vi "CalculateAverages.vi"(6 "Settings":T1={"Name of test"="", "Date"=timestamp(0 s since 1904-01-01), "Location"="", "Template"="", "Soundcard"="", "resolution"=32, "Sampling rate"=48000, "Ch1 Gain "=25.0, "Ch2 Gain"=10.0, "Sample time (s)"=0.3, "Pre-trigger (s)"=0.01, "Hammer Threshold"=10.0, "Positions"=12, "Taps/Position"=5, "Set Names"="", "Freq resolution"=10.0, "Hammer cutoff"=0.0, "Mic cutoff"=0.0, "Double bounce "=0.0, "Hammer Cal"=10.0, "dB Offset"=0.0, "Accel Cal"=10.0, "Vibrometer Cal"=0.0, "Mic Cal"=0.0, "Output"=2, "Voltage Cal"=1.0, "Vibrometer Port"="ASRL27::INSTR", "Range"=4, "High Pass"=2, "Bandwidth"=4, "X Range"=[], "Y Range"=[], "dB Spread"=0.0, "Trigger"=0, "Ch_1"=25, "Ch_2"=25, "flip?"=FALSE, "60Hz"=FALSE, "Time offset"=0.0, "Piezo Cal"=1.0, "Default Notes"=""} {"Ch_2" min=1 step=1; "Ch_1" min=1 max=100 step=1; "Trigger" items=["Hammer (force)", "Self-tap", "Spacebar"]; "Bandwidth" items=["1 kHz"=1, "5 kHz"=5, "10 kHz"=10, "25 kHz"=25, "50 kHz"=50, "100 kHz"=100]; "High Pass" items=["Off", "13 Hz", "104 Hz"]; "Range" items=["10 mm/s"=1, "20 mm/s"=2, "50 mm/s"=5, "100 mm/s"=10, "200 mm/s"=20, "500 mm/s"=50, "1 m/s"=100, "2 m/s"=200]; "Output" items=["Accelerometer", "Speed (from acceleration)", "Microphone", "Vibrometer", "Piezo"]; "Voltage Cal" format="%#_13g"; "Ch2 Gain" format="%#_13g"; "Ch1 Gain" format="%#_13g"; "Double bounce" min=0.0; "Mic cutoff" min=0.0 format="%#_4g"; "Hammer cutoff" min=0.0 format="%#_4g"; "Freq resolution" min=0.0; "Pre-trigger (s)" format="%#_13g"; "Date" format="%<%H:%M\n%d/%m/%y>T"; "resolution" items=["16 bit"=16, "24 bit"=24, "32 bit"=32]; "Sampling rate" items=["22050 samp/s"=22050, "44100 samp/s"=44100, "48000 samp/s"=48000]}, 8 "Task":enum16{"Set", "Test"}(ring), 10 "Inst:Test Name":string, 11 "Last Data File":path) -> ()   [LabVIEW 2022 SP3]
uses:
  PreferencesControl.ctl
panel:
  # "Hz"
  # "dB"
  # "dB"
  # "sec"
  # "sec"
  # "mV/Pa"
  # "mV/m/s2"
  # "mV/mm/s"
  # "V/N"
  # "sec"
  # "sec"
  # "mV/N"
  # "a.u."
  # "a.u."
  # "sec"
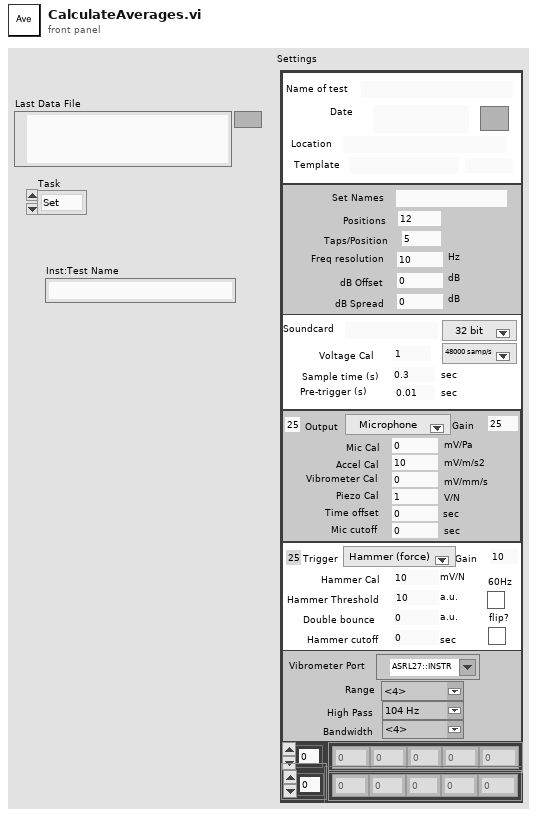
[diagram p1: front panel]
types:
  T1 = typedef "PreferencesControl.ctl" = cluster{"Name of test":string, "Date":timestamp, "Location":string, "Template":string, "Soundcard":string, "resolution":u16, "Sampling rate":u16, "Ch1 Gain ":dbl, "Ch2 Gain":dbl, "Sample time (s)":dbl, "Pre-trigger (s)":dbl, "Hammer Threshold":dbl, "Positions":i16, "Taps/Position":i16, "Set Names":string, "Freq resolution":dbl, "Hammer cutoff":dbl, "Mic cutoff":dbl, "Double bounce ":dbl, "Hammer Cal":dbl, "dB Offset":dbl, "Accel Cal":dbl, "Vibrometer Cal":dbl, "Mic Cal":dbl, "Output":u16, "Voltage Cal":dbl, "Vibrometer Port":refnum<visa-resource-name>, "Range":u16, "High Pass":u16, "Bandwidth":u16, "X Range":cluster{"Minimum":dbl, "Maximum":dbl, "Increment":dbl, "Minor Increment":dbl, "Start":dbl}[], "Y Range":cluster{"Minimum":dbl, "Maximum":dbl, "Increment":dbl, "Minor Increment":dbl, "Start":dbl}[], "dB Spread":dbl, "Trigger":u16, "Ch_1":u8, "Ch_2":u8, "flip?":bool, "60Hz":bool, "Time offset":dbl, "Piezo Cal":dbl, "Default Notes":string}
  T2 = cluster{"Test":string, "Set":string, "Position":string, "Tap":string}
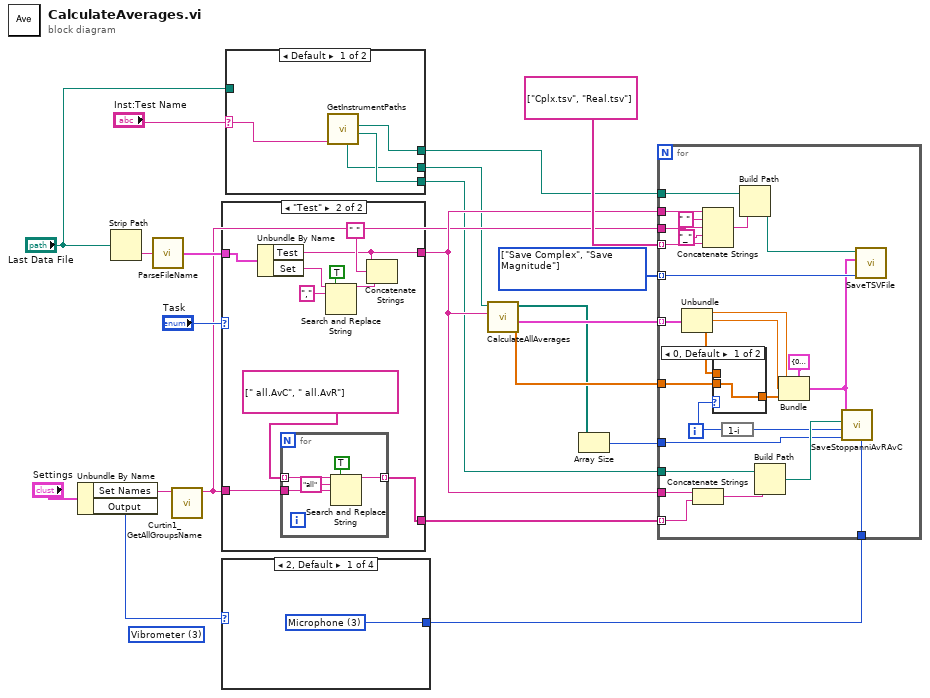
[diagram p0: block diagram]
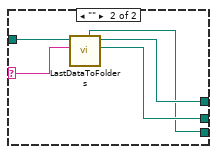
[diagram p2: hidden frame]
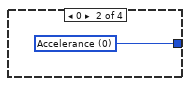
[diagram p3: hidden frame]
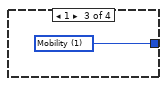
[diagram p4: hidden frame]
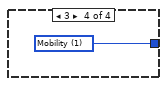
[diagram p5: hidden frame]
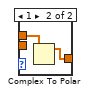
[diagram p6: hidden frame]
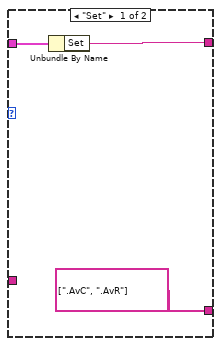
[diagram p7: hidden frame]
diagram:
  w7 = enum16{"Save Magnitude", "Save Complex"}[] [enum."Save Complex", enum."Save Magnitude"] items=["Save Magnitude", "Save Complex"]
  (unwired) u16 3 items=["Acclerometer", "Displacement", "Microphone", "Vibrometer"] ("Channel 1")
  n1 = Unbundle By Name("Settings") -> ("Set Names"=w12:string, "Output"=w9:u16)
  n2 = Strip Path(path="Last Data File") -> (name=w21:string)  [unwired: 1 out]
  n3 = call "ParseFileName.vi"("String in"=w21) -> ("Name"=w18:T2)  [unwired: 2 out]
  n4 = call "Curtin1_GetAllGroupsName.vi"("Set Names in"=w12) -> ("Set Names out"=w6:string)  [unwired: 10 in]
  n5 = case shown="\"Test\"" "Task" {
    tunnel: w18 -> [w24 w34]
    tunnel: [w23 w28] -> w15
    tunnel: [string[] [".AvC", ".AvR"] w26] -> w14
    tunnel: w6 -> [_ w25]
    frame "Set" {
      n6 = Unbundle By Name(w24) -> ("Set"=w23:string)
    }
    frame "Test" {
      n7 = Unbundle By Name(w34) -> ("Test"=w28:string, "Set"=w32:string)
      n8 = for {
        tunnel: string[] [" all.AvC", " all.AvR"] -> [w38] mode=indexing
        tunnel: [w37] -> w26 mode=indexing
        tunnel: w25 -> [w35]
        n9 = Search and Replace String(replace all?=TRUE ("replace all? (F)"), input string=w38, search string="all", replace string=w35) -> (result string=w37:string)  [unwired: 4 in, 3 out]
      }
      n10 = Search and Replace String(replace all?=TRUE ("replace all? (F)"), input string=w32, search string=",") -> (result string=w30:string)  [unwired: 5 in, 3 out]
      n11 = Concatenate Strings(w28, " " ("string"), w30) -> ()  [unwired: 1 out]
    }
  }
  n12 = case shown="2, Default" w9 {
    tunnel: [w40 w41 w42 w43] -> w8
    frame 2, Default {
      w40 = u8 3 items=["Accelerance", "Mobility", "Receptance", "Microphone", "Unknown"] ("dtAccel")
    }
    frame 0 {
      w41 = u8 0 items=["Accelerance", "Mobility", "Receptance", "Microphone", "Unknown"] ("dtAccel")
    }
    frame 1 {
      w42 = u8 1 items=["Accelerance", "Mobility", "Receptance", "Microphone", "Unknown"] ("dtAccel")
    }
    frame 3 {
      w43 = u8 1 items=["Accelerance", "Mobility", "Receptance", "Microphone", "Unknown"] ("dtAccel")
    }
  }
  n13 = case shown="Default" "Inst:Test Name" {
    selector: "Inst:Test Name" -> [w44 w51]
    tunnel: [w47 w48] -> w5
    tunnel: [w46 w50] -> w4
    tunnel: [w45 w49] -> w3
    tunnel: "Last Data File" -> [_ w52]
    frame Default {
      n14 = call "GetInstrumentPaths.vi"("Instrument"=w44) -> ("Path To Test Folder"=w47:path, "Path to csv Folder"=w46:path, "Path To TRF Folder"=w45:path)  [unwired: 6 in, 2 out]
    }
    frame "" {
      n15 = call "LastDataToFolders.vi"("Inst:Test Name"=w51, "Last Path"=w52) -> ("Path To TRF Folder"=w49:path, "Path to csv Folder"=w50:path, "Path to test Folder"=w48:path)  [unwired: 7 in]
    }
  }
  n16 = call "CalculateAllAverages.vi"("Instrument"=w15, "Path To TRF Folder"=w3) -> ("Complex Average"=w16:cdb[], "FRF Spectra"=w17:cluster{dbl, "df":dbl, "FFT {X}":dbl[]}[], "Array"=w11:path[])  [unwired: 7 in]
  n17 = Array Size(array=w11) -> (size(s)=w10:i32)
  n18 = for {
    tunnel: string[] ["Cplx.tsv", "Real.tsv"] -> [w78] mode=indexing
    tunnel: w15 -> [w75]
    tunnel: w4 -> [w62]
    tunnel: w17 -> [w60] mode=indexing
    tunnel: w16 -> [w70]
    tunnel: w5 -> [w68]
    tunnel: w15 -> [w66]
    tunnel: w14 -> [w63] mode=indexing
    tunnel: w10 -> [w59]
    tunnel: w8 -> [w58]
    tunnel: w7 -> [w56] mode=indexing
    tunnel: w6 -> [w55]
    i -> [w57]
    n19 = Unbundle(w60) -> (w73:dbl, "df"=w72:dbl, "FFT {X}"=w69:dbl[])
    n20 = Concatenate Strings(w66, w63) -> (w65:string)
    n21 = Concatenate Strings(w75, " " ("string"), w55, "_" ("format string"), w78) -> (w77:string)
    n22 = case shown="0, Default" w57 {
      tunnel: [w79 w80] -> w71
      tunnel: w70 -> [w79 _]
      tunnel: w69 -> [_ w81]
      frame 0, Default {
      }
      frame 1 {
        n23 = Complex To Polar(r * e^(i*theta)=w81) -> (r=w80:dbl[])  [unwired: 1 out]
      }
    }
    n24 = expression code="1-i"(w57) -> (w64:i32)
    n25 = Build Path(base path=w62, name or relative path=w77) -> (appended path=w61:path)
    n26 = Build Path(base path=w68, name or relative path=w65) -> (appended path=w67:path)
    n27 = Bundle(cluster=cluster{"t0":dbl, "dt":dbl, "Y":cdb[]} {"t0"=0.0, "dt"=0.0, "Y"=[]} ("Complex FRF"), "t0"=w73, "dt"=w72, "Y"=w71) -> (w53:cluster{"t0":dbl, "dt":dbl, "Y":cdb[]})
    n28 = call "SaveStoppanniAvRAvC.vi"("dtAccel"=w58, "nAverages"=w59, "fComplex"=w64, "file (use dialog)"=w67, "Complex FRF"=w53) -> ()  [unwired: 6 in, 1 out]
    n29 = call "SaveTSVFile.vi"("Task"=w56, "FRF"=w53, "Path"=w61) -> ()  [unwired: 8 in, 1 out]
  }
